vi "Generate Code From DAQ Assistant.vi"() -> ()   [LabVIEW 2020]
panel:
  out "Waveform Chart":dynamicdata(graph)
  in  "stop":bool
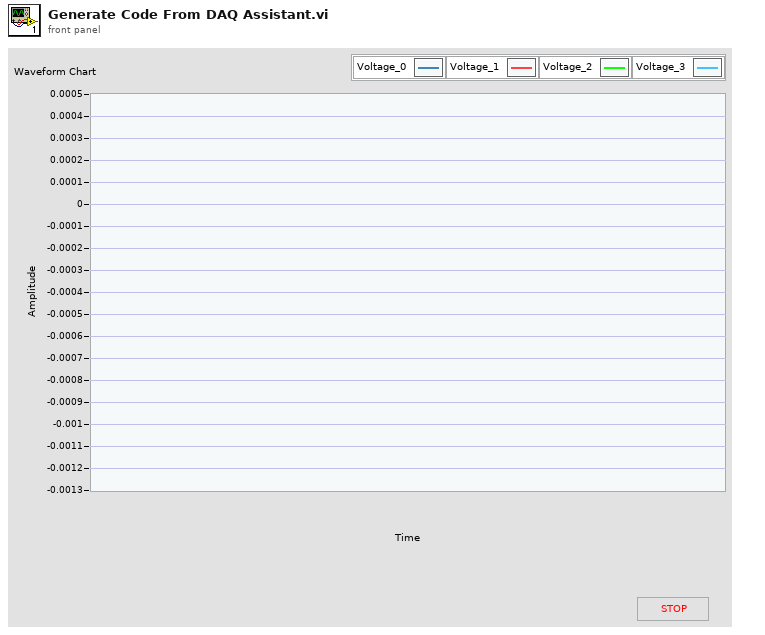
[diagram p1: front panel]
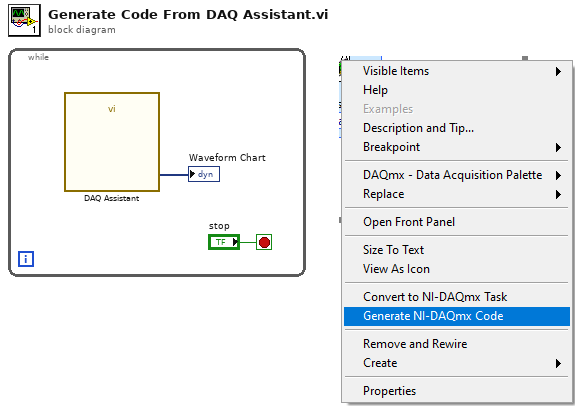
[diagram p0: block diagram]
diagram:
  n1 = while {
    stop <- "stop" stop-if-true
    n2 = call "DAQ Assistant"() -> ("data"=→"Waveform Chart":dynamicdata)  [unwired: 16 in, 3 out]
  }
